vi "1 port_Save Sweep Data to csv.vi"(3 "Meas Type":string="QuickView_", 4 "PostTest Capacitance":dbl[](array[numeric]), 5 "Selected Exp Settings":T5={"Floor_Sweep_Stop_V"=36.0, "Resistance Threshold"=1.0, "Floor_Sweep_Start_V"=36.0, "Floor_Sweep_Step_V"=1.0, "Roof_Sweep_Stop_V"=36.0, "Roof_Sweep_Start_V"=36.0, "Roof_Sweep_Step_V"=1.0, "Experiment Name"="", "Meas_Type"=[0, 2, 4]}, 6 "PreTest Capacitance":dbl[](array[numeric]), 7 "Filepath":path, 9 "ks5080A_Meaurements":T4, 10 "Date Cluster":T3, 11 "Test Information":T2={"Exp Name"="Cold Switching", "Lot"="0233A", "Wafer"="15", "Die Type"="L22", "Die X "="6", "Die Y"="8", "Exp"="1", "Die X_Y"="8"}) -> ()   [LabVIEW 2013]
uses:
  Controls/Date Control.ctl
  Controls/Test Information.ctl
  Controls/ks5080A_Measurements.ctl
  Controls/Individual User Inputs_MultiTest.ctl
  Controls/Test Selection.ctl
  <vilib>/Utility/file.llb/Write To Spreadsheet File (string).vi
panel:
  in  "Tab Control":T1(tab)
  # "Calculation Settings"
  # "Test Settings"
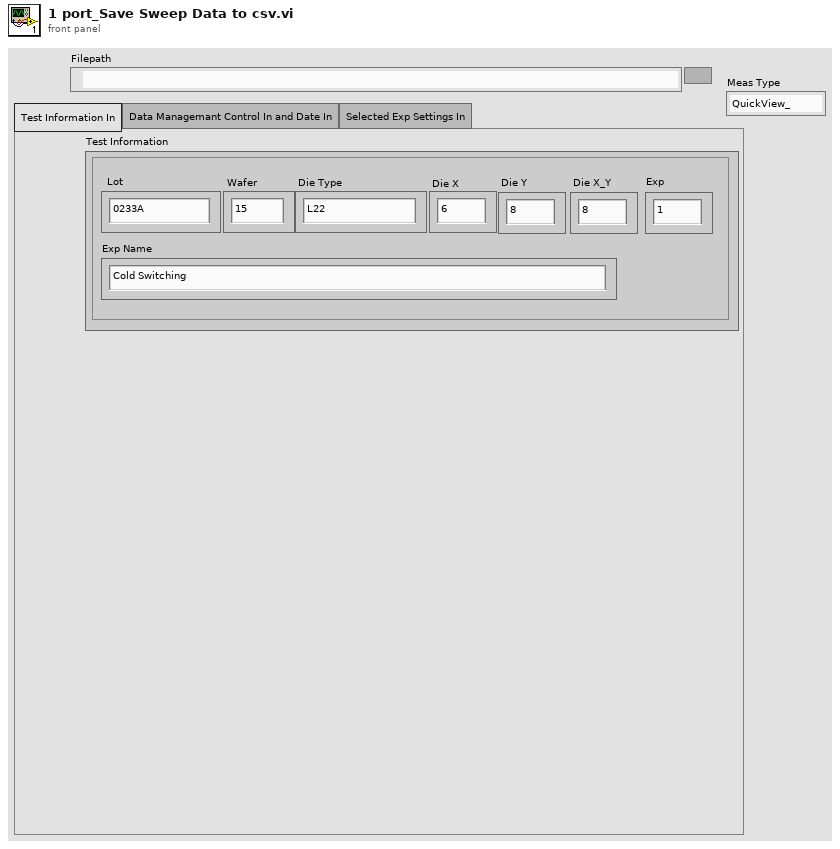
[diagram p1: front panel]
types:
  T1 = enum32{"Test Information In", "Data Managemant Control In and Date In", "Selected Exp Settings In"}
  T2 = typedef "Test Information.ctl" = cluster{"Exp Name":string, "Lot":string, "Wafer":string, "Die Type":string, "Die X ":string, "Die Y":string, "Exp":string, "Die X_Y":string}
  T3 = typedef "Date Control.ctl" = cluster{"Date":string, "Start Time":string, "Stop Time":string}
  T4 = typedef "ks5080A_Measurements.ctl" = cluster{"Bias_Sweep_Setting":dbl[], "Bias_voltage measurements":dbl[], "Bias_current measurements":dbl[], "P1_Capacitance":dbl[], "P2_Capacitance":dbl[], "DMM_Measurement_V":dbl[], "Contact_Source Current measurements":dbl[], "Contact_Sink Current measurements":dbl[], "Calculated_Resistance":dbl[], "P3_Capacitance":dbl[], "Port 1_S_parm":string[], "Port 2_S_parm":string[], "Port 3_S_parm":string[]}
  T5 = typedef "Individual User Inputs_MultiTest.ctl" = cluster{"Floor_Sweep_Stop_V":dbl, "Resistance Threshold":dbl, "Floor_Sweep_Start_V":dbl, "Floor_Sweep_Step_V":dbl, "Roof_Sweep_Stop_V":dbl, "Roof_Sweep_Start_V":dbl, "Roof_Sweep_Step_V":dbl, "Experiment Name":string, "Meas_Type":T6}
  T6 = typedef "Test Selection.ctl" = i32[]
  T7 = enum16{"open", "replace", "create", "open or create", "replace or create", "replace or create with confirmation"}
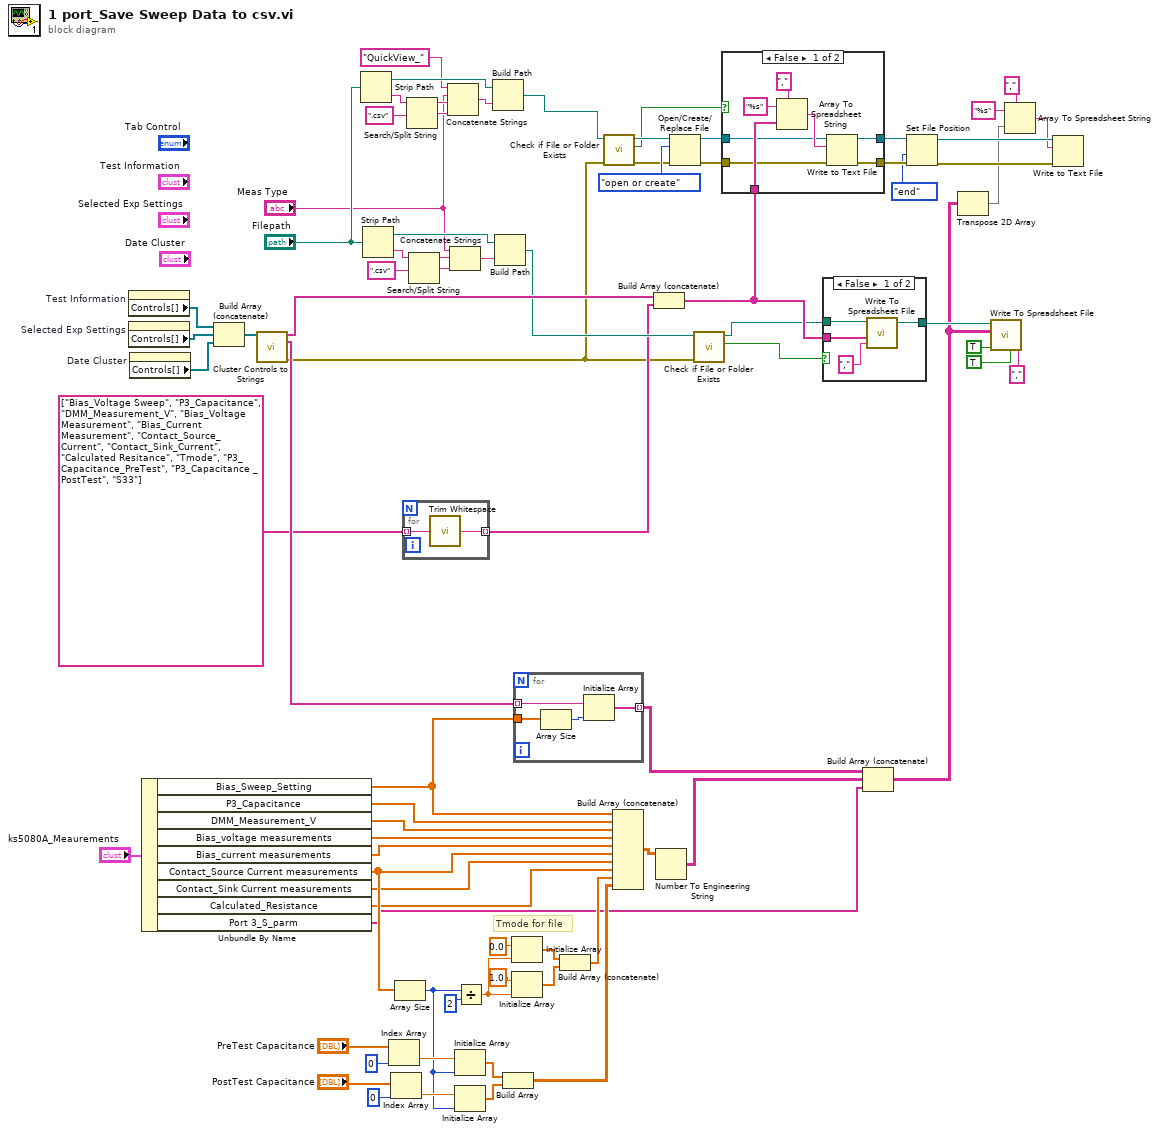
[diagram p0: block diagram]
diagram:
  # "Tmode for file"
  n1 = property on="Test Information" class="Clust (strict)"() -> ("Controls[]"=w79:refnum<vi>[])  [unwired: 2 in, 2 out]
  n2 = property on="Selected Exp Settings" class="Clust (strict)"() -> ("Controls[]"=w7:refnum<vi>[])  [unwired: 2 in, 2 out]
  n3 = property on="Date Cluster" class="Clust (strict)"() -> ("Controls[]"=w1:refnum<vi>[])  [unwired: 2 in, 2 out]
  n4 = Unbundle By Name("ks5080A_Meaurements") -> ("Bias_Sweep_Setting"=w57:dbl[], "P3_Capacitance"=w73:dbl[], "DMM_Measurement_V"=w72:dbl[], "Bias_voltage measurements"=w71:dbl[], "Bias_current measurements"=w70:dbl[], "Contact_Source Current measurements"=w69:dbl[], "Contact_Sink Current measurements"=w35:dbl[], "Calculated_Resistance"=w34:dbl[], "Port 3_S_parm"=w15:string[])
  n5 = Build Array (concatenate)(w79, w7, w1) -> (w78:refnum<vi>[])
  n6 = call "Cluster Controls to Strings.vi"("Controls[]"=w78) -> ("Control Labels"=w58:string[], "Control Values"=w77:string[], "Error Out"=w2:errorcluster)  [unwired: 12 in]
  n7 = Strip Path(path="Filepath") -> (stripped path=w52:path, name=w55:string)
  n8 = Strip Path(path="Filepath") -> (stripped path=w18:path, name=w21:string)
  n9 = Index Array(array="PreTest Capacitance", index=0) -> (element=w30:dbl)
  n10 = Index Array(array="PostTest Capacitance", index=0) -> (element=w29:dbl)
  n11 = Array Size(array=w69) -> (size(s)=w28:i32)
  n12 = for {
    tunnel: string[] ["Bias_Voltage Sweep", "P3_Capacitance", "DMM_Measurement_V", "Bias_Voltage Measurement", "Bias_Current Measurement", "Contact_Source_Current", "Contact_Sink_Current", "Calculated Resitance", "Tmode", "P3_Capacitance_PreTest", "P3_Capacitance _PostTest", "S33"] -> [w81] mode=indexing
    tunnel: [w80] -> w3 mode=indexing
    n13 = call <vilib>:"Trim Whitespace.vi"("string"=w81) -> ("trimmed string"=w80:string)  [unwired: 1 in]
  }
  n14 = Search/Split String(string=w55, search string/char (-)=".csv" ("search string")) -> (substring before match=w50:string, match + rest of string=w53:string)  [unwired: 1 in, 1 out]
  n15 = Search/Split String(string=w21, search string/char (-)=".csv" ("search string")) -> (substring before match=w16:string, match + rest of string=w19:string)  [unwired: 1 in, 1 out]
  n16 = Concatenate Strings("QuickView_" ("search string"), "Meas Type", w50, w53) -> (w51:string)
  n17 = Concatenate Strings("Meas Type", w16, w19) -> (w17:string)
  n18 = Initialize Array(w30, w28) -> (w27:dbl[])
  n19 = Initialize Array(w29, w28) -> (w26:dbl[])
  n20 = Divide(x=w28, y=2) -> (x/y=w75:dbl)
  n21 = Build Path(base path=w52, name or relative path=w51) -> (appended path=w13:path)
  n22 = Build Path(base path=w18, name or relative path=w17) -> (appended path=w9:path)
  n23 = Build Array(w27, w26) -> (w25:dbl[][])
  n24 = Initialize Array(0.0, w75) -> (w76:dbl[])
  n25 = Initialize Array(1.0, w75) -> (w66:dbl[])
  n26 = for {
    tunnel: w57 -> [w85]
    tunnel: w77 -> [w84] mode=indexing
    tunnel: [w82] -> w61 mode=indexing
    n27 = Array Size(array=w85) -> (size(s)=w83:i32)
    n28 = Initialize Array(w84, w83) -> (w82:string[])
  }
  n29 = Build Array (concatenate)(w76, w66) -> (w33:dbl[])
  n30 = call <vilib>:"Check if File or Folder Exists.vi"("error in (no error)"=w2, "path"=w13) -> ("error out"=w14:errorcluster, "file or folder exists?"=w11:bool, "dup path"=w12:path)  [unwired: 7 in]
  n31 = Build Array (concatenate)(w57, w73, w72, w71, w70, w69, w35, w34, w33, w25) -> (w59:dbl[][])
  n32 = Build Array (concatenate)(w58, w3) -> (w48:string[])
  n33 = Number To Engineering String(4:w59) -> (0:w60:string[][])  [unwired: 3 in]
  n34 = Open/Create/Replace File(file path (use dialog)=w12, error in=w14, operation (0:open)=T7."open or create") -> (refnum out=w47:refnum<file>, error out=w46:errorcluster)  [unwired: 3 in, 1 out]
  n35 = call <vilib>:"Check if File or Folder Exists.vi"("error in (no error)"=w2, "path"=w9) -> ("file or folder exists?"=w49:bool, "dup path"=w8:path)  [unwired: 7 in, 1 out]
  n36 = case shown="False" w11 {
    tunnel: w48 -> [w91 _]
    tunnel: w47 -> [w89 w95]
    tunnel: w46 -> [w88 w94]
    tunnel: [w87 w94] -> w44
    tunnel: [w86 w95] -> w45
    frame False {
      n37 = Array To Spreadsheet String(delimiter (Tab)="," ("delimiter (\\t)"), array=w91, 3:"%s" ("format string")) -> (spreadsheet string=w90:string)
      n38 = Write to Text File(file (use dialog)=w89, text=w90, error in=w88) -> (refnum out=w86:refnum<file>, error out=w87:errorcluster)  [unwired: 1 in, 1 out]
    }
    frame True {
    }
  }
  n39 = case shown="False" w49 {
    tunnel: w8 -> [w99 w100]
    tunnel: w48 -> [w98 _]
    tunnel: [w96 w100] -> w65
    frame False {
      n40 = call-poly <vilib>:"Write To Spreadsheet File.vi"("delimiter (\\t)"="," ("delimiter (\\t)"), "1D data"=w98, "file path (dialog if empty)"=w99) -> ("new file path (Not A Path if cancelled)"=w96:path)  [unwired: 5 in]
    }
    frame True {
    }
  }
  n41 = Build Array (concatenate)(w61, w60, w15) -> (w37:string[][])
  n42 = Set File Position(refnum=w45, from (0:start)=enum16{"start", "end", "current"}."end", error in=w44) -> (refnum out=w39:refnum<file>, error out=w40:errorcluster)  [unwired: 1 in]
  n43 = Transpose 2D Array(2D array=w37) -> (transposed array=w36:string[][])
  n44 = call-poly <vilib>:"Write To Spreadsheet File.vi"("delimiter (\\t)"="," ("delimiter (\\t)"), "transpose? (no:F)"=TRUE, "append to file? (new file:F)"=TRUE, "2D data"=w37, "file path (dialog if empty)"=w65) -> ()  [unwired: 3 in, 1 out]
  n45 = Array To Spreadsheet String(delimiter (Tab)="," ("delimiter (\\t)"), array=w36, 3:"%s" ("format string")) -> (spreadsheet string=w38:string)
  n46 = Write to Text File(file (use dialog)=w39, text=w38, error in=w40) -> ()  [unwired: 1 in, 3 out]
